vi "Write Index of Plugin.vi"(8 "error in (no error)":errorcluster, 10 "Index of Plugin":i32, 11 "Plugin Display UI in":refnum<class "Plugin Display UI.lvclass">) -> (0 "error out":errorcluster, 3 "Plugin Display UI out":refnum<class "Plugin Display UI.lvclass">)   [LabVIEW 2011, in "Plugin Display UI.lvclass"]
uses:
  Plugin Display UI.lvclass
  Plugin Display UI.lvclass/Plugin Display UI.ctl
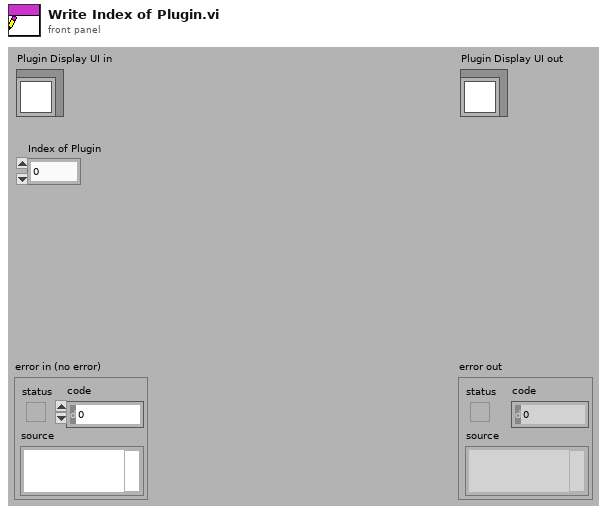
[diagram p1: front panel]
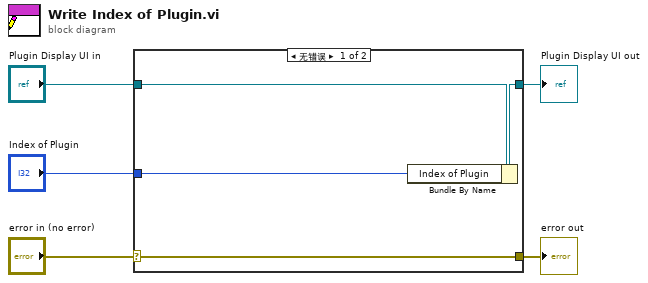
[diagram p0: block diagram]
diagram:
  n1 = case shown="无错误" "error in (no error)" {
    selector: "error in (no error)" -> [w9 w10]
    tunnel: [w9 w10] -> w4
    tunnel: [w7 w11] -> w2
    tunnel: "Plugin Display UI in" -> [w8 w11]
    tunnel: "Index of Plugin" -> [w6 _]
    frame No Error {
      n2 = Bundle By Name(cluster=w8, "Index of Plugin"=w6) -> (w7:refnum<class "Plugin Display UI.lvclass">)
    }
    frame Error {
    }
  }
  "error out" <- w4
  "Plugin Display UI out" <- w2
